vi "Safety_Check.vi"(1 "Adam Loop Count":i32, 2 "Ch Names":string[](array[string]), 3 "Values":dbl[](array[numeric]) format="%.2f") -> (0 "Scan comment":string)   [LabVIEW 2010]
uses:
  ADAM Client/Sub VIs/ADAM Controls/Update_scan_value.ctl
  Anemometry/Anemometry Sub Vis/Globals/Gas_management_global.vi
  ADAM_Global.vi
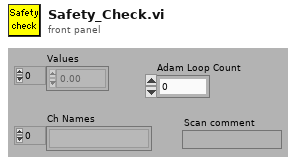
[diagram p1: front panel]
types:
  T1 = cluster{"Channel name":string, "Set value of A to":dbl, "Set value of B to":dbl, "Set value of C to":dbl, "Set value of D to":dbl}
  T2 = typedef "Update_scan_value.ctl" = cluster{"Channel Name":string, "New Value":dbl}
  T3 = enum16{"Append to Global", "Read Global then Clear"}
  T4 = enum16{"On", "Off", "Always On", "Always Off", "Delete"}
  T5 = typedef "LVDateTimeRec.ctl" = cluster{"fractional second":dbl, "second":i32, "minute":i32, "hour":i32, "day of month":i32, "month":i32, "year":i32, "day of week":i32, "day of year":i32, "DST":i32}
  T6 = cluster{"Channel name":string, "Set value of A to":dbl, "Set value of B to":dbl, "Set value of C to":dbl, "Set value of D to":dbl}[]
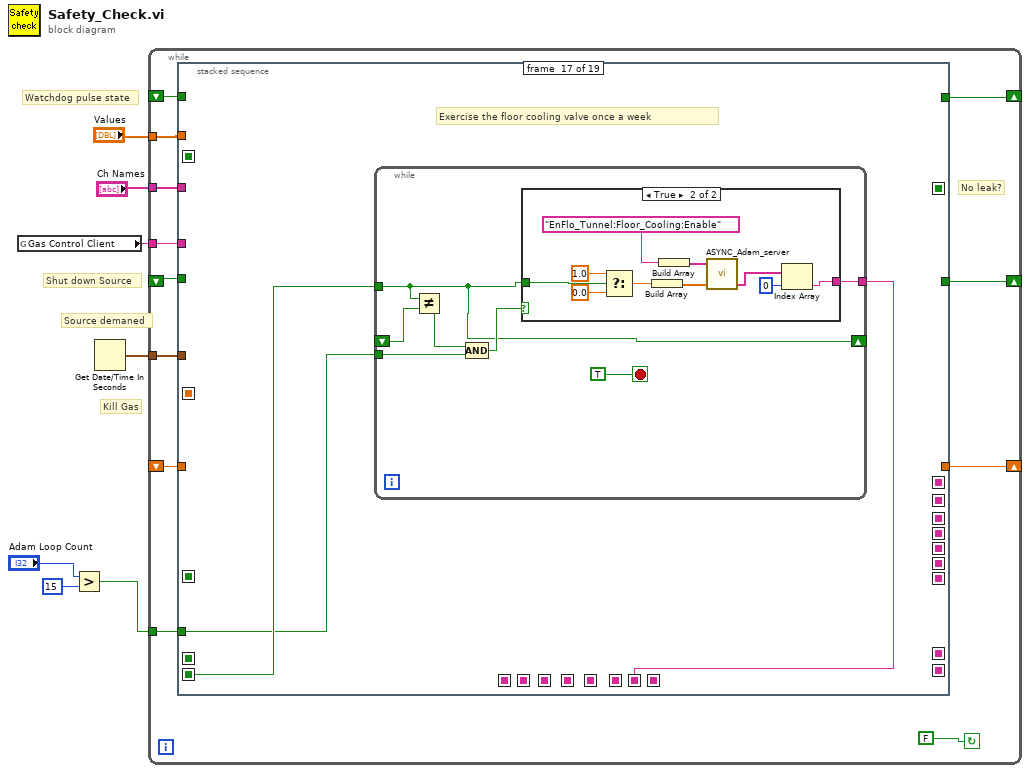
[diagram p0: block diagram]
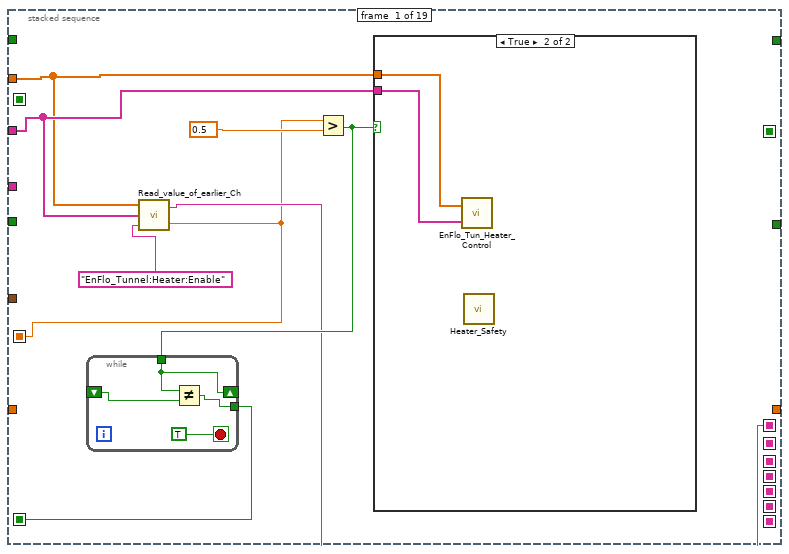
[diagram p2: hidden frame]
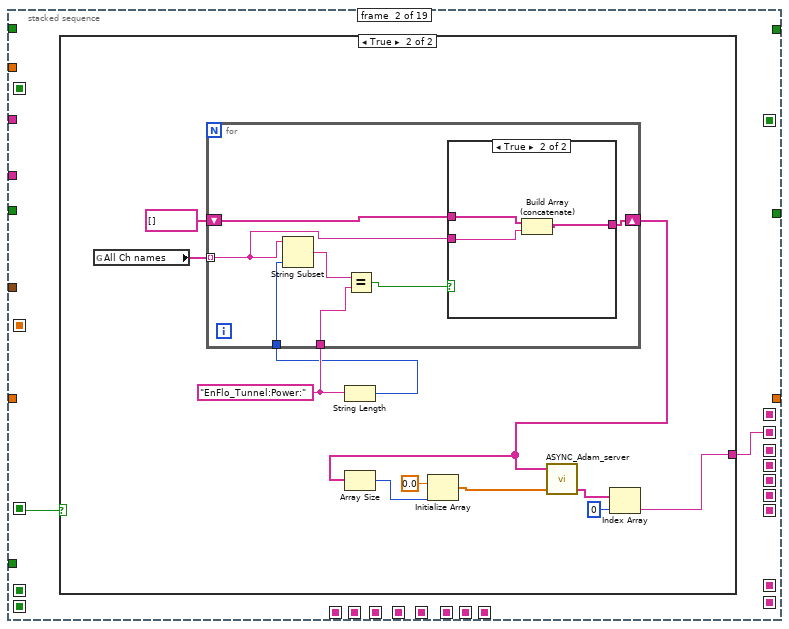
[diagram p4: hidden frame]
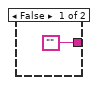
[diagram p5: hidden frame]
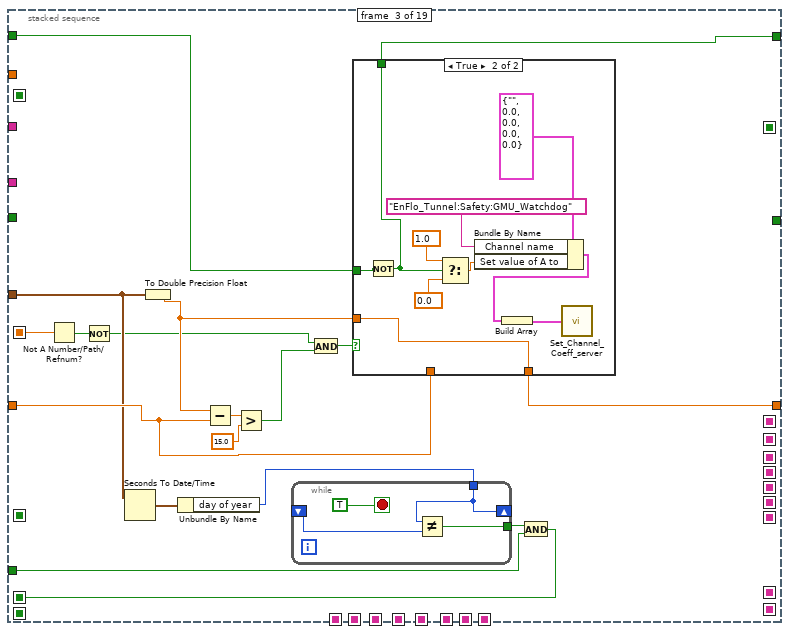
[diagram p7: hidden frame]
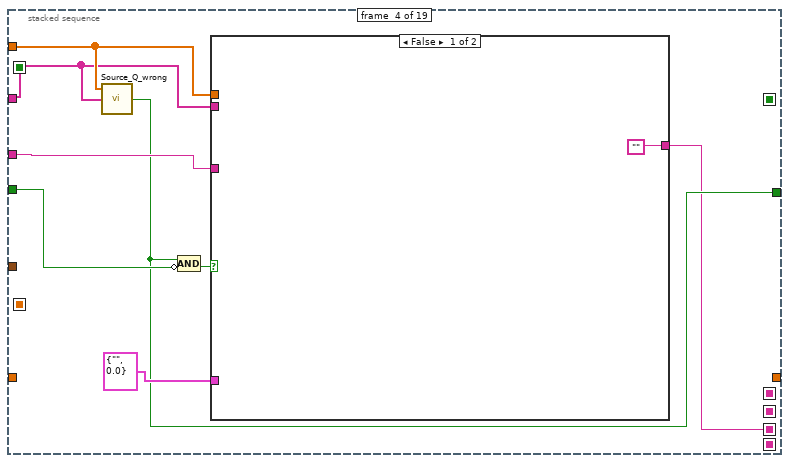
[diagram p9: hidden frame]
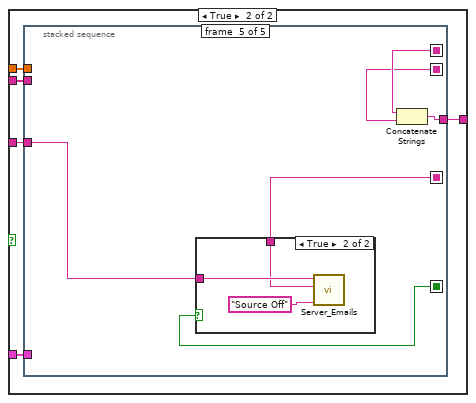
[diagram p10: hidden frame]
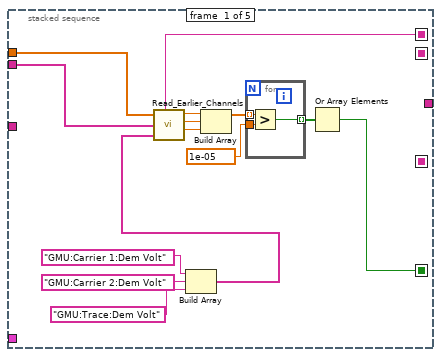
[diagram p11: hidden frame]
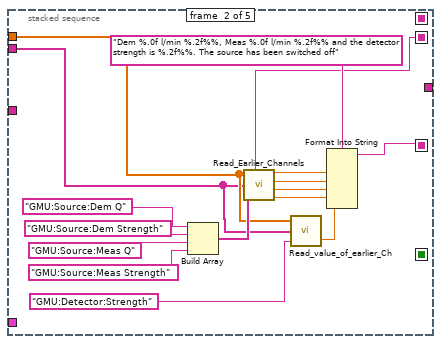
[diagram p12: hidden frame]
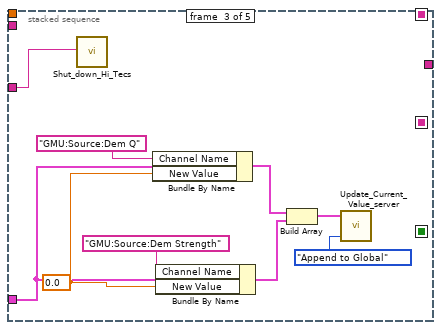
[diagram p13: hidden frame]
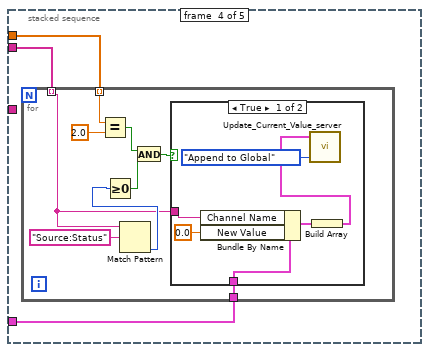
[diagram p14: hidden frame]
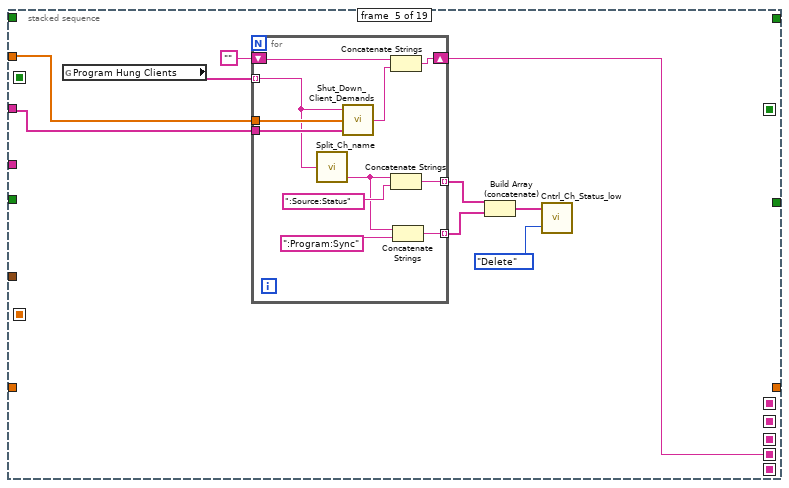
[diagram p17: hidden frame]
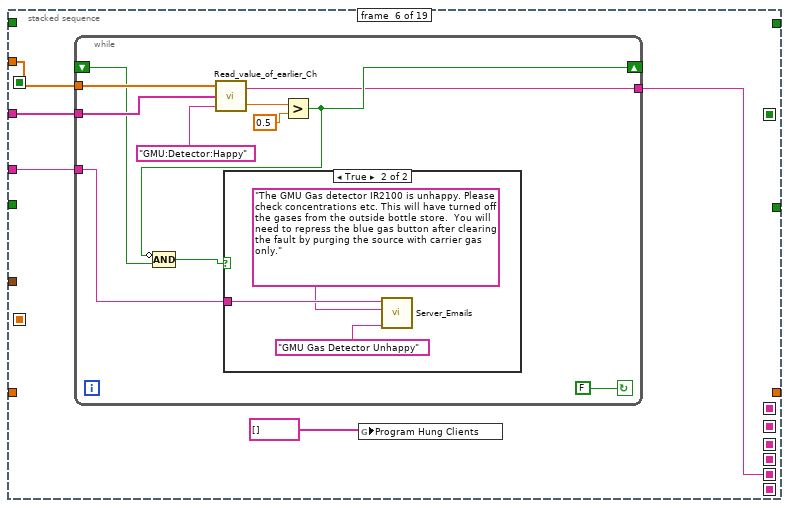
[diagram p18: hidden frame]
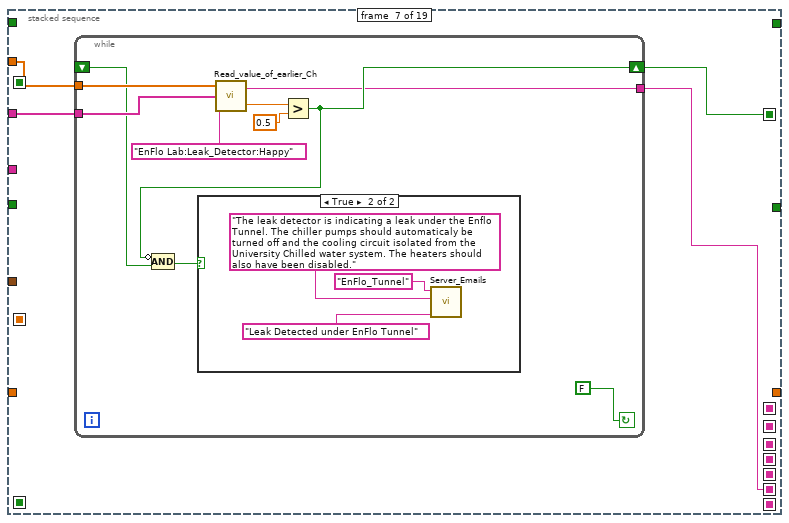
[diagram p20: hidden frame]
diagram:
  # "Shut down Source"
  # "Source demaned"
  # "Watchdog pulse state"
  # "Kill Gas"
  n1 = global read "Gas_management_global.vi" "Gas Control Client"() -> (w5:string)
  n2 = Greater?(x="Adam Loop Count", y=15) -> (0:w2:bool)
  n3 = Get Date/Time In Seconds() -> (seconds since 1Jan1904=w1:timestamp)
  n4 = while {
    shift-left: _ -> [w14]
    shift-right: [w13] -> _
    shift-left: _ -> [w16]
    shift-right: [w15] -> _
    tunnel: w5 -> [w18]
    tunnel: "Ch Names" -> [w19]
    tunnel: "Values" -> [w17]
    shift-right: [w11] -> _
    shift-left: _ -> [w10]
    tunnel: w2 -> [w9]
    tunnel: w1 -> [w8]
    stop <- FALSE continue-if-true
    # "No leak?"
    n5 = stacked-sequence {
      seq-local: [_ _ _ _ _ _ w216 _ _ _ _ _ _ _ _ _ _ _ _] -> [_ _ _ _ _ _ _ _ _ _ w308 _ _ _ _ _ _ _ _]
      seq-local: [w22 _ _ _ _ _ _ _ _ _ _ _ _ _ _ _ _ _ _] -> [_ w35 _ _ _ _ _ _ _ _ _ _ _ _ _ _ _ _ _]
      seq-local: [_ _ w65 _ _ _ _ _ _ _ _ _ _ _ _ _ _ _ _] -> [_ _ _ _ _ _ _ _ _ _ _ _ _ _ _ _ _ _ _]
      seq-local: [_ _ _ _ _ _ _ _ _ _ _ _ w368 _ _ _ _ _ _] -> [_ _ _ _ _ _ _ _ _ _ _ _ _ w386 _ _ _ _ _]
      seq-local: [_ _ _ _ _ _ _ _ _ _ _ _ _ w378 _ _ _ _ _] -> [_ _ _ _ _ _ _ _ _ _ _ _ _ _ _ _ w510 _ _]
      seq-local: [w21 _ _ _ _ _ _ _ _ _ _ _ _ _ _ _ _ _ _] -> [_ _ _ _ _ _ _ _ _ _ _ _ _ _ _ _ _ _ w597]
      seq-local: [_ w34 _ _ _ _ _ _ _ _ _ _ _ _ _ _ _ _ _] -> [_ _ _ _ _ _ _ _ _ _ _ _ _ _ _ _ _ _ w596]
      seq-local: [_ _ _ w93 _ _ _ _ _ _ _ _ _ _ _ _ _ _ _] -> [_ _ _ _ _ _ _ _ _ _ _ _ _ _ _ _ _ _ w595]
      seq-local: [_ _ _ _ w176 _ _ _ _ _ _ _ _ _ _ _ _ _ _] -> [_ _ _ _ _ _ _ _ _ _ _ _ _ _ _ _ _ _ w594]
      seq-local: [_ _ _ _ _ w196 _ _ _ _ _ _ _ _ _ _ _ _ _] -> [_ _ _ _ _ _ _ _ _ _ _ _ _ _ _ _ _ _ w593]
      seq-local: [_ _ _ _ _ _ w215 _ _ _ _ _ _ _ _ _ _ _ _] -> [_ _ _ _ _ _ _ _ _ _ _ _ _ _ _ _ _ _ w592]
      seq-local: [_ _ _ _ _ _ _ w232 _ _ _ _ _ _ _ _ _ _ _] -> [_ _ _ _ _ _ _ _ _ _ _ _ _ _ _ _ _ _ w591]
      seq-local: [_ _ _ _ _ _ _ _ w264 _ _ _ _ _ _ _ _ _ _] -> [_ _ _ _ _ _ _ _ _ _ _ _ _ _ _ _ _ _ w581]
      seq-local: [_ _ _ _ _ _ _ _ _ w284 _ _ _ _ _ _ _ _ _] -> [_ _ _ _ _ _ _ _ _ _ _ _ _ _ _ _ _ _ w580]
      seq-local: [_ _ _ _ _ _ _ _ _ _ w305 _ _ _ _ _ _ _ _] -> [_ _ _ _ _ _ _ _ _ _ _ _ _ _ _ _ _ _ w583]
      seq-local: [_ _ _ _ _ _ _ _ _ _ _ w333 _ _ _ _ _ _ _] -> [_ _ _ _ _ _ _ _ _ _ _ _ _ _ _ _ _ _ w584]
      seq-local: [_ _ _ _ _ _ _ _ _ _ _ _ w356 _ _ _ _ _ _] -> [_ _ _ _ _ _ _ _ _ _ _ _ _ _ _ _ _ _ w585]
      seq-local: [_ _ _ _ _ _ _ _ _ _ _ _ _ w375 _ _ _ _ _] -> [_ _ _ _ _ _ _ _ _ _ _ _ _ _ _ _ _ _ w586]
      seq-local: [_ _ _ _ _ _ _ _ _ _ _ _ _ _ w443 _ _ _ _] -> [_ _ _ _ _ _ _ _ _ _ _ _ _ _ _ _ _ _ w587]
      seq-local: [_ _ _ _ _ _ _ _ _ _ _ _ _ _ _ w472 _ _ _] -> [_ _ _ _ _ _ _ _ _ _ _ _ _ _ _ _ _ _ w588]
      seq-local: [_ _ _ _ _ _ _ _ _ _ _ _ _ _ _ _ w508 _ _] -> [_ _ _ _ _ _ _ _ _ _ _ _ _ _ _ _ _ _ w589]
      seq-local: [_ _ _ _ _ _ _ _ _ _ _ _ _ _ _ _ _ w529 _] -> [_ _ _ _ _ _ _ _ _ _ _ _ _ _ _ _ _ _ w590]
      seq-local: [w20 _ _ _ _ _ _ _ _ _ _ _ _ _ _ _ _ _ _] -> [_ _ w63 _ _ _ _ _ _ _ _ _ _ _ _ _ _ _ _]
      tunnel: w19 -> [w25 _ _ w95 w183 w198 w217 w233 w265 w286 w306 w339 w364 w387 w448 w475 _ w536 _]
      tunnel: w18 -> [_ _ _ w100 _ w197 _ _ _ _ _ _ _ _ _ _ _ _ _]
      tunnel: w17 -> [w24 _ _ w96 w179 w199 w218 w234 w266 w287 w307 w340 w365 w388 w449 w476 _ w535 _]
      tunnel: w16 -> [_ _ w76 _ _ _ _ _ _ _ _ _ _ _ _ _ _ _ _]
      tunnel: [_ _ w75 _ _ _ _ _ _ _ _ _ _ _ _ _ _ _ _] -> w15
      tunnel: w14 -> [_ _ _ w99 _ _ _ _ _ _ _ _ _ _ _ _ _ _ _]
      tunnel: [_ _ _ w94 _ _ _ _ _ _ _ _ _ _ _ _ _ _ _] -> w13
      tunnel: [_ _ w74 _ _ _ _ _ _ _ _ _ _ _ _ _ _ _ _] -> w11
      tunnel: w10 -> [_ _ w70 _ _ _ _ _ _ _ _ _ _ _ _ _ _ _ _]
      tunnel: w9 -> [_ _ w66 _ _ _ _ _ _ w285 _ _ _ w379 w444 _ w509 w530 _]
      tunnel: w8 -> [_ _ w64 _ _ _ _ _ _ _ _ _ _ _ _ _ _ _ _]
      frame #0 {
        n6 = call "Read_value_of_earlier_Ch.vi"("Desired Ch to Read"="EnFlo_Tunnel:Heater:Enable", "Ch names"=w25, "Present scan array"=w24) -> ("Value"=w20:dbl, "Scan comment"=w21:string)  [unwired: 1 in]
        n7 = Greater?(x=w20, y=0.5) -> (0:w23:bool)
        n8 = while {
          shift-right: [w31] -> _
          shift-left: _ -> [w30]
          tunnel: w23 -> [w31]
          tunnel: [w28] -> w22
          stop <- TRUE stop-if-true
          n9 = Not Equal?(x=w31, y=w30) -> (x != y?=w28:bool)
        }
        n10 = case shown="True" w23 {
          tunnel: w24 -> [_ w33]
          tunnel: w25 -> [_ w32]
          frame False {
          }
          frame True {
            n11 = call "EnFlo_Tun_Heater_Control.vi"("Ch Names"=w32, "Values"=w33) -> ()  [unwired: 1 out]
            n12 = call "Heater_Safety.vi"() -> ()  [unwired: 3 in, 5 out]
          }
        }
      }
      frame #1 {
        n13 = case shown="True" w35 {
          tunnel: ["" w38] -> w34
          frame False {
          }
          frame True {
            w47 = "EnFlo_Tunnel:Power:"
            n14 = global read "ADAM_Global.vi" "All Ch names"() -> (w37:string[])
            n15 = String Length(string=w47) -> (length=w46:i32)
            n16 = for {
              shift-right: [w49] -> w42
              shift-left: string[] [] -> [w50]
              tunnel: w37 -> [w53] mode=indexing
              tunnel: w46 -> [w54]
              tunnel: w47 -> [w51]
              n17 = String Subset(string=w53, length (rest)=w54) -> (substring=w52:string)  [unwired: 1 out]
              n18 = Equal?(x=w52, y=w51) -> (x = y?=w48:bool)
              n19 = case shown="True" w48 {
                tunnel: w53 -> [_ w58]
                tunnel: w50 -> [w55 w56]
                tunnel: [w55 w57] -> w49
                frame False {
                }
                frame True {
                  n20 = Build Array (concatenate)(w56, w58) -> (w57:string[])
                }
              }
            }
            n21 = Array Size(array=w42) -> (size(s)=w43:i32)
            n22 = Initialize Array(0.0 ("element"), w43) -> (w41:dbl[])
            n23 = call "ASYNC_Adam_server.vi"("Values"=w41, "Channel Names"=w42) -> ("Scan Comments"=w40:string[])  [unwired: 1 in, 2 out]
            n24 = Index Array(array=w40, index=0) -> (element=w38:string)
          }
        }
      }
      frame #2 {
        n25 = Not A Number/Path/Refnum?(number/path/refnum=w63) -> (NaN/Path/Refnum?=w62:bool)
        n26 = Not(x=w62) -> (.not. x?=w60:bool)
        n27 = Seconds To Date/Time(time stamp (now)=w64) -> (date time rec=w69:T5)  [unwired: 1 in]
        n28 = To Double Precision Float(number=w64) -> (double precision float=w73:dbl)
        n29 = Unbundle By Name(w69) -> ("day of year"=w68:i32)
        n30 = Subtract(x=w73, y=w70) -> (x-y=w72:dbl)
        n31 = Greater?(x=w72, y=15.0) -> (0:w61:bool)
        n32 = while {
          shift-right: [w80] -> _
          shift-left: _ -> [w79]
          tunnel: w68 -> [w80]
          tunnel: [w78] -> w67
          stop <- TRUE stop-if-true
          n33 = Not Equal?(x=w80, y=w79) -> (x != y?=w78:bool)
        }
        n34 = And(x=w60, y=w61) -> (x .and. y?=w59:bool)
        n35 = case shown="True" w59 {
          tunnel: w76 -> [w81 w85]
          tunnel: [w81 w84] -> w75
          tunnel: [w82 w83] -> w74
          tunnel: w73 -> [_ w83]
          tunnel: w70 -> [w82 _]
          frame False {
          }
          frame True {
            n36 = Not(x=w85) -> (.not. x?=w84:bool)
            n37 = Select(t=1.0 ("Suction"), s=w84, f=0.0 ("Suction")) -> (s? t:f=w88:dbl)
            n38 = Bundle By Name(cluster=T1 {"Channel name"="", "Set value of A to"=0.0, "Set value of B to"=0.0, "Set value of C to"=0.0, "Set value of D to"=0.0}, "Channel name"="EnFlo_Tunnel:Safety:GMU_Watchdog" ("Desired Ch to Read"), "Set value of A to"=w88) -> (w92:T1)
            n39 = Build Array(w92) -> (w87:T6)
            n40 = call "Set_Channel_Coeff_server.vi"("Set Array"=w87) -> ()
          }
        }
        n41 = And(x=w67, y=w66) -> (x .and. y?=w65:bool)
      }
      frame #3 {
        n42 = call "Source_Q_wrong.vi"("Ch Names"=w95, "Values"=w96) -> ("Gas Error?"=w94:bool)  [unwired: 1 out]
        n43 = Compound Arithmetic op=AND(w94, invert w99) -> (w98:bool)
        n44 = case shown="False" w98 {
          tunnel: w100 -> [_ w106]
          tunnel: w96 -> [_ w105]
          tunnel: w95 -> [_ w104]
          tunnel: T2 {"Channel Name"="", "New Value"=0.0} ("Update Scan Value Cluster") -> [_ w103]
          tunnel: ["" w102] -> w93
          frame False {
          }
          frame True {
            n45 = stacked-sequence {
              seq-local: [_ w138 _ _ _] -> [_ _ _ _ w171]
              seq-local: [w108 _ _ _ _] -> [_ _ _ _ w170]
              seq-local: [w107 _ _ _ _] -> [_ _ _ _ w169]
              seq-local: [_ w124 _ _ _] -> [_ _ _ _ w168]
              tunnel: w106 -> [_ _ w141 _ w172]
              tunnel: w105 -> [w118 w128 _ w150 _]
              tunnel: w104 -> [w119 w127 _ w151 _]
              tunnel: w103 -> [_ _ w140 w149 _]
              tunnel: [_ _ _ _ w167] -> w102
              frame #0 {
                n46 = Build Array("GMU:Carrier 1:Dem Volt", "GMU:Carrier 2:Dem Volt", "GMU:Trace:Dem Volt") -> (w120:string[])
                n47 = call "Read_Earlier_Channels.vi"("Present scan array"=w118, "Ch names"=w119, "Desired Channels"=w120) -> ("Scan comments"=w107:string, "Index 0"=w114:dbl, "Index 1"=w113:dbl, "Index 2"=w112:dbl)  [unwired: 2 out]
                n48 = Build Array(w114, w113, w112) -> (w111:dbl[])
                n49 = for {
                  tunnel: w111 -> [w123] mode=indexing
                  tunnel: 1e-05 -> [w122]
                  tunnel: [w121] -> w109 mode=indexing
                  n50 = Greater?(x=w123, y=w122) -> (0:w121:bool)
                }
                n51 = Or Array Elements(Boolean array=w109) -> (logical OR=w108:bool)
              }
              frame #1 {
                n52 = Build Array("GMU:Source:Dem Q", "GMU:Source:Dem Strength", "GMU:Source:Meas Q", "GMU:Source:Meas Strength") -> (w133:string[])
                n53 = call "Read_Earlier_Channels.vi"("Present scan array"=w128, "Ch names"=w127, "Desired Channels"=w133) -> ("Scan comments"=w124:string, "Index 0"=w132:dbl, "Index 1"=w131:dbl, "Index 2"=w130:dbl, "Index 3"=w129:dbl)  [unwired: 1 out]
                n54 = call "Read_value_of_earlier_Ch.vi"("Desired Ch to Read"="GMU:Detector:Strength", "Ch names"=w127, "Present scan array"=w128) -> ("Value"=w125:dbl)  [unwired: 1 in, 1 out]
                n55 = Format Into String(format string="Dem %.0f l/min %.2f%%, Meas %.0f l/min %.2f%% and the detector strength is %.2f%%. The source has been switched off" ("Format String"), w132, w131, w130, w129, w125) -> (resulting string=w138:string)  [unwired: 2 in, 1 out]
              }
              frame #2 {
                w142 = 0.0 ("Bundle Element")
                n56 = call "Shut_down_Hi_Tecs.vi"("Client Name"=w141) -> ()  [unwired: 6 out]
                n57 = Bundle By Name(cluster=w140, "Channel Name"="GMU:Source:Dem Q", "New Value"=w142) -> (w147:T2)
                n58 = Bundle By Name(cluster=w140, "Channel Name"="GMU:Source:Dem Strength", "New Value"=w142) -> (w148:T2)
                n59 = Build Array(w147, w148) -> (w144:T2[])
                n60 = call "Update_Current_Value_server.vi"("Mode"=T3."Append to Global", "Update array in"=w144) -> ()  [unwired: 1 in, 1 out]
              }
              frame #3 {
                n61 = for {
                  tunnel: w151 -> [w152] mode=indexing
                  tunnel: w150 -> [w158] mode=indexing
                  tunnel: w149 -> [w153]
                  n62 = Equal?(x=w158, y=2.0) -> (x = y?=w155:bool)
                  n63 = Match Pattern(string=w152, regular expression="Source:Status") -> (offset past match=w159:i32)  [unwired: 4 out]
                  n64 = Greater Or Equal To 0?(x=w159) -> (x >= 0?=w156:bool)
                  n65 = And(x=w155, y=w156) -> (x .and. y?=w154:bool)
                  n66 = case shown="True" w154 {
                    tunnel: w153 -> [w166 _]
                    tunnel: w152 -> [w165 _]
                    frame True {
                      n67 = Bundle By Name(cluster=w166, "Channel Name"=w165, "New Value"=0.0) -> (w163:T2)
                      n68 = Build Array(w163) -> (w162:T2[])
                      n69 = call "Update_Current_Value_server.vi"("Mode"=T3."Append to Global", "Update array in"=w162) -> ()  [unwired: 1 in, 1 out]
                    }
                    frame False {
                    }
                  }
                }
              }
              frame #4 {
                n70 = case shown="True" w170 {
                  tunnel: w172 -> [_ w175]
                  tunnel: w171 -> [_ w174]
                  frame False {
                  }
                  frame True {
                    n71 = call "Server_Emails.vi"("Client Name Contains"=w175, "Message"=w174, "Subject"="Source Off") -> ()  [unwired: 2 in, 3 out]
                  }
                }
                n72 = Concatenate Strings(w169, w168) -> (w167:string)
              }
            }
          }
        }
      }
      frame #4 {
        n73 = global read "ADAM_Global.vi" "Program Hung Clients"() -> (w184:string[])
        n74 = for {
          tunnel: w184 -> [w193] mode=indexing
          tunnel: w179 -> [w195]
          tunnel: w183 -> [w194]
          tunnel: [w191] -> w182 mode=indexing
          tunnel: [w188] -> w181 mode=indexing
          shift-right: [w186] -> w176
          shift-left: "" -> [w187]
          n75 = call "Split_Ch_name.vi"("Ch name"=w193) -> ("Low level"=w190:string)  [unwired: 2 out]
          n76 = call "Shut_Down_Client_Demands.vi"("Ch Names"=w194, "Values"=w195, "Client Name"=w193) -> ("Comments"=w185:string)
          n77 = Concatenate Strings(w187, w185) -> (w186:string)
          n78 = Concatenate Strings(w190, ":Source:Status") -> (w191:string)
          n79 = Concatenate Strings(w190, ":Program:Sync") -> (w188:string)
        }
        n80 = Build Array (concatenate)(w182, w181) -> (w180:string[])
        n81 = call "Cntrl_Ch_Status_low.vi"("Mode"=T4."Delete", "Channel names"=w180) -> ()  [unwired: 1 out]
      }
      frame #5 {
        n82 = while {
          tunnel: w199 -> [w211]
          tunnel: w198 -> [w210]
          shift-right: [w205] -> _
          shift-left: _ -> [w206]
          tunnel: w197 -> [w203]
          tunnel: [w201] -> w196
          stop <- FALSE continue-if-true
          n83 = call "Read_value_of_earlier_Ch.vi"("Desired Ch to Read"="GMU:Detector:Happy", "Ch names"=w210, "Present scan array"=w211) -> ("Value"=w208:dbl, "Scan comment"=w201:string)  [unwired: 1 in]
          n84 = Greater?(x=w208, y=0.5) -> (0:w205:bool)
          n85 = Compound Arithmetic op=AND(invert w205, w206) -> (w204:bool)
          n86 = case shown="True" w204 {
            tunnel: w203 -> [_ w213]
            frame False {
            }
            frame True {
              n87 = call "Server_Emails.vi"("Client Name Contains"=w213, "Message"="The GMU Gas detector IR2100 is unhappy. Please check concentrations etc. This will have turned off the gases from the outside bottle store.  You will need to repress the blue gas button after clearing the fault by purging the source with carrier gas only.", "Subject"="GMU Gas Detector Unhappy") -> ()  [unwired: 2 in, 3 out]
            }
          }
        }
        n88 = global write "ADAM_Global.vi" "Program Hung Clients"(string[] [] ("Program Hung Clients")) -> ()
      }
      frame #6 {
        n89 = while {
          tunnel: w218 -> [w228]
          tunnel: w217 -> [w227]
          shift-right: [w222] -> w216
          shift-left: _ -> [w223]
          tunnel: [w219] -> w215
          stop <- FALSE continue-if-true
          n90 = call "Read_value_of_earlier_Ch.vi"("Desired Ch to Read"="EnFlo Lab:Leak_Detector:Happy", "Ch names"=w227, "Present scan array"=w228) -> ("Value"=w225:dbl, "Scan comment"=w219:string)  [unwired: 1 in]
          n91 = Greater?(x=w225, y=0.5) -> (0:w222:bool)
          n92 = Compound Arithmetic op=AND(invert w222, w223) -> (w221:bool)
          n93 = case shown="True" w221 {
            frame False {
            }
            frame True {
              n94 = call "Server_Emails.vi"("Client Name Contains"="EnFlo_Tunnel", "Message"="The leak detector is indicating a leak under the Enflo Tunnel. The chiller pumps should automaticaly be turned off and the cooling circuit isolated from the  University Chilled water system. The heaters should also have been disabled.", "Subject"="Leak Detected under EnFlo Tunnel") -> ()  [unwired: 2 in, 3 out]
            }
          }
        }
      }
      frame #7 {
        n95 = while {
          tunnel: w234 -> [w250]
          tunnel: w233 -> [w249]
          shift-right: [w243] -> _
          shift-left: _ -> [w239]
          tunnel: [w235] -> w232
          stop <- FALSE continue-if-true
          w241 = 60.0 ("y")
          n96 = Decrement(x=w241) -> (x-1=w242:dbl)
          n97 = Select(t=w242, s=w239, f=w241) -> (s? t:f=w240:dbl)
          n98 = call "Read_value_of_earlier_Ch.vi"("Desired Ch to Read"="EnFlo_Tunnel:Chilled Water:Motor1 Temp", "Ch names"=w249, "Present scan array"=w250) -> ("Value"=w257:dbl, "Scan comment"=w237:string)  [unwired: 1 in]
          n99 = call "Read_value_of_earlier_Ch.vi"("Desired Ch to Read"="EnFlo_Tunnel:Chilled Water:Motor2 Temp", "Ch names"=w249, "Present scan array"=w250) -> ("Value"=w254:dbl, "Scan comment"=w236:string)  [unwired: 1 in]
          n100 = Greater?(x=w257, y=w240) -> (0:w251:bool)
          n101 = Greater?(x=w254, y=w240) -> (0:w252:bool)
          n102 = Or(x=w251, y=w252) -> (x .or. y?=w245:bool)
          n103 = call "Read_value_of_earlier_Ch.vi"("Desired Ch to Read"="EnFlo_Tunnel:Chiller_Pump:Enable", "Ch names"=w249, "Present scan array"=w250) -> ("Value"=w247:dbl, "Scan comment"=w238:string)  [unwired: 1 in]
          n104 = Greater?(x=w247, y=0.5) -> (0:w244:bool)
          n105 = And(x=w244, y=w245) -> (x .and. y?=w243:bool)
          n106 = Compound Arithmetic op=AND(w243, invert w239) -> (w256:bool)
          n107 = case shown="False" w256 {
            tunnel: w241 -> [_ w260]
            frame False {
            }
            frame True {
              n108 = Format Into String(format string="The Chilled Water Motor Temp is greater than %.0f deg C." ("Message"), w260) -> (resulting string=w259:string)  [unwired: 2 in, 1 out]
              n109 = call "Server_Emails.vi"("Client Name Contains"="EnFlo_Tunnel", "Message"=w259, "Subject"="Chilled Water Motor Temp") -> ()  [unwired: 2 in, 3 out]
            }
          }
          n110 = Concatenate Strings(w238, w237, w236) -> (w235:string)
        }
      }
      frame #8 {
        n111 = while {
          tunnel: w266 -> [w280]
          tunnel: w265 -> [w279]
          shift-right: [w268] -> _
          shift-left: _ -> [w274]
          shift-left: _ -> [w273]
          shift-left: _ -> [w272]
          tunnel: [w267] -> w264
          stop <- FALSE continue-if-true
          n112 = call "Read_value_of_earlier_Ch.vi"("Desired Ch to Read"="FFID:System:Enable", "Ch names"=w279, "Present scan array"=w280) -> ("Value"=w275:dbl, "Scan comment"=w267:string)  [unwired: 1 in]
          n113 = Greater?(x=w275, y=0.5) -> (0:w268:bool)
          n114 = Compound Arithmetic op=AND(w268, w274, invert w273, invert w272) -> (w270:bool)
          n115 = Compound Arithmetic op=AND(invert w268, invert w274, w273, w272) -> (w271:bool)
          n116 = Or(x=w270, y=w271) -> (x .or. y?=w269:bool)
          n117 = case shown="True" w269 {
            tunnel: w275 -> [_ w281]
            tunnel: w268 -> [_ _]
            frame False {
            }
            frame True {
              n118 = Build Array(w281) -> (w283:dbl[])
              n119 = call "ASYNC_Adam_server.vi"("Values"=w283, "Channel Names"=string[] ["GMU:Gas:Enable"]) -> ()  [unwired: 1 in, 3 out]
            }
          }
        }
      }
      frame #9 {
        # "Resetting A Tunnel speed to zero if the drive in turned off\nso that the belts do not slip when the tunnel is turned on again."
        n120 = while {
          tunnel: w287 -> [w300]
          tunnel: w286 -> [w299]
          shift-right: [w291] -> _
          shift-left: _ -> [w294]
          shift-left: _ -> [w293]
          shift-left: _ -> [w292]
          tunnel: w285 -> [w290]
          tunnel: [w288] -> w284
          stop <- FALSE continue-if-true
          n121 = call "Read_value_of_earlier_Ch.vi"("Desired Ch to Read"="A_Tunnel:Motor:Enable", "Ch names"=w299, "Present scan array"=w300) -> ("Value"=w295:dbl, "Scan comment"=w288:string)  [unwired: 1 in]
          n122 = Less?(x=w295, y=0.5) -> (x < y?=w291:bool)
          n123 = Compound Arithmetic op=AND(w291, w294, invert w293, invert w292, w290) -> (w289:bool)
          n124 = case shown="True" w289 {
            tunnel: w291 -> [_ _]
            frame False {
            }
            frame True {
              w303 = string[] ["A_Tunnel:Speed:Dem Velocity", "A_Tunnel:Speed:Dem Voltage"] ("Channel Names")
              n125 = Array Size(array=w303) -> (size(s)=w304:i32)
              n126 = Initialize Array(0.0 ("element"), w304) -> (w302:dbl[])
              n127 = call "ASYNC_Adam_server.vi"("Values"=w302, "Channel Names"=w303) -> ()  [unwired: 1 in, 3 out]
            }
          }
        }
      }
      frame #10 {
        n128 = case shown="True" w308 {
          tunnel: w307 -> [w313 _]
          tunnel: w306 -> [w312 _]
          tunnel: [w309 ""] -> w305
          frame False {
            n129 = for {
              tunnel: w313 -> [w323]
              tunnel: w312 -> [w322]
              tunnel: string[] ["EnFlo_Tunnel:Heater:Enable", "EnFlo_Tunnel:Chiller_Pump:Enable", "EnFlo_Tunnel:Tap_Water:Enable"] ("Ch Names") -> [w318] mode=indexing
              shift-right: [w316] -> w309
              shift-left: "" -> [w317]
              n130 = call "Read_value_of_earlier_Ch.vi"("Desired Ch to Read"=w318, "Ch names"=w322, "Present scan array"=w323) -> ("Value"=w320:dbl, "Scan comment"=w315:string)  [unwired: 1 in]
              n131 = Greater?(x=w320, y=0.5) -> (0:w319:bool)
              n132 = case shown="False" w319 {
                tunnel: w318 -> [_ w328]
                tunnel: ["" w325] -> w314
                frame False {
                }
                frame True {
                  n133 = Build Array(w328) -> (w331:string[])
                  n134 = Build Array(0.0) -> (w330:dbl[])
                  n135 = call "ASYNC_Adam_server.vi"("Values"=w330, "Channel Names"=w331) -> ("Scan Comments"=w326:string[])  [unwired: 1 in, 2 out]
                  n136 = Index Array(array=w326, index=0) -> (element=w325:string)
                }
              }
              n137 = Concatenate Strings(w317, w315, w314) -> (w316:string)
            }
          }
          frame True {
          }
        }
      }
      frame #11 {
        w341 = "EnFlo_Tunnel:Heater:Enable" ("Ch Name")
        n138 = call "Read_value_of_earlier_Ch.vi"("Desired Ch to Read"=w341, "Ch names"=w339, "Present scan array"=w340) -> ("Value"=w346:dbl, "Scan comment"=w335:string)  [unwired: 1 in]
        n139 = call "Read_value_of_earlier_Ch.vi"("Desired Ch to Read"="EnFlo_Tunnel:Reference:Velocity", "Ch names"=w339, "Present scan array"=w340) -> ("Value"=w343:dbl, "Scan comment"=w334:string)  [unwired: 1 in]
        n140 = Greater?(x=w346, y=0.5) -> (0:w338:bool)
        n141 = Less?(x=w343, y=0.25) -> (x < y?=w342:bool)
        n142 = And(x=w338, y=w342) -> (x .and. y?=w337:bool)
        n143 = case shown="False" w337 {
          tunnel: w341 -> [_ w352]
          tunnel: ["" w349] -> w336
          frame False {
          }
          frame True {
            n144 = Build Array(w352) -> (w355:string[])
            n145 = Build Array(0.0) -> (w354:dbl[])
            n146 = call "ASYNC_Adam_server.vi"("Values"=w354, "Channel Names"=w355) -> ("Scan Comments"=w350:string[])  [unwired: 1 in, 2 out]
            n147 = Index Array(array=w350, index=0) -> (element=w349:string)
          }
        }
        n148 = Concatenate Strings(w335, w334, w336) -> (w333:string)
      }
      frame #12 {
        n149 = call "Read_value_of_earlier_Ch.vi"("Desired Ch to Read"="EnFlo_Tunnel:Chiller_Pump:Running", "Ch names"=w364, "Present scan array"=w365) -> ("Value"=w366:dbl, "Scan comment"=w359:string)  [unwired: 1 in]
        n150 = call "Read_value_of_earlier_Ch.vi"("Desired Ch to Read"="Uni:Chilled Water:Temp", "Ch names"=w364, "Present scan array"=w365) -> ("Value"=w361:dbl, "Scan comment"=w358:string)  [unwired: 1 in]
        n151 = call "Read_value_of_earlier_Ch.vi"("Desired Ch to Read"="EnFlo_Tunnel:Reference:Velocity", "Ch names"=w364, "Present scan array"=w365) -> ("Value"=w360:dbl, "Scan comment"=w357:string)  [unwired: 1 in]
        n152 = Less?(x=w361, y=20.0) -> (x < y?=w371:bool)
        n153 = Greater?(x=w360, y=0.4) -> (0:w372:bool)
        n154 = Greater?(x=w366, y=0.5) -> (0:w374:bool)
        n155 = Compound Arithmetic op=AND(w374, w371, w372) -> (w368:bool)
        n156 = Concatenate Strings(w359, w358, w357) -> (w356:string)
      }
      frame #13 {
        w384 = "EnFlo_Tunnel:Heat_Ex_Div_Valve:Dem Pos"
        n157 = case shown="False" w386 {
          tunnel: w388 -> [_ w426]
          tunnel: w387 -> [_ w427]
          tunnel: w384 -> [_ w430]
          tunnel: [0.0 ("upper limit") w436] -> w380
          tunnel: ["" w421] -> w377
          frame False {
          }
          frame True {
            n158 = call "Read_value_of_earlier_Ch.vi"("Desired Ch to Read"="EnFlo_Tunnel:Exit Duct:Dem Temp", "Ch names"=w427, "Present scan array"=w426) -> ("Value"=w435:dbl, "Scan comment"=w425:string)  [unwired: 1 in]
            n159 = call "Read_value_of_earlier_Ch.vi"("Desired Ch to Read"="EnFlo_Tunnel:Exit Duct Top:Temp", "Ch names"=w427, "Present scan array"=w426) -> ("Value"=w431:dbl, "Scan comment"=w424:string)  [unwired: 1 in]
            n160 = call "Read_value_of_earlier_Ch.vi"("Desired Ch to Read"="EnFlo_Tunnel:Exit Duct:Temp", "Ch names"=w427, "Present scan array"=w426) -> ("Value"=w432:dbl, "Scan comment"=w423:string)  [unwired: 1 in]
            n161 = call "Read_value_of_earlier_Ch.vi"("Desired Ch to Read"=w430, "Ch names"=w427, "Present scan array"=w426) -> ("Value"=w433:dbl, "Scan comment"=w422:string)  [unwired: 1 in]
            n162 = Add(x=w431, y=w432) -> (x+y=w440:dbl)
            n163 = Divide(x=w440, y=2.0) -> (x/y=w442:dbl)
            n164 = Concatenate Strings(w425, w424, w423, w422) -> (w421:string)
            n165 = call "Back_End_Chiller_PID.vi"("Present Value"=w442, "Previous Control Sum"=w433, "Setpoint"=w435) -> ("Dem Output"=w439:dbl)
            n166 = In Range and Coerce(upper limit=100.0, x=w439, lower limit=0.0) -> (coerced(x)=w436:dbl)  [unwired: 1 out]
          }
        }
        n167 = while {
          shift-right: [w418] -> w385
          shift-left: _ -> [_]
          tunnel: w386 -> [w418]
          shift-left: _ -> [_]
          shift-left: _ -> [_]
          shift-left: _ -> [_]
          shift-left: _ -> [_]
          shift-left: _ -> [_]
          shift-left: _ -> [_]
          shift-left: _ -> [_]
          shift-left: _ -> [_]
          shift-left: _ -> [_]
          shift-left: _ -> [_]
          shift-left: _ -> [_]
          shift-left: _ -> [_]
          shift-left: _ -> [_]
          shift-left: _ -> [_]
          shift-left: _ -> [_]
          shift-left: _ -> [_]
          shift-left: _ -> [w417]
          tunnel: [w417] -> w383
          stop <- TRUE stop-if-true
        }
        n168 = And(x=w385, y=w383) -> (x .and. y?=w382:bool)
        n169 = case shown="False" w382 {
          tunnel: [w390 w401] -> w381
          tunnel: w380 -> [_ w401]
          tunnel: [w389 FALSE] -> w378
          frame False {
            # "Exercise valve once a week"
            n170 = Seconds To Date/Time() -> (date time rec=w391:T5)  [unwired: 2 out]
            n171 = Unbundle By Name(w391) -> ("day of week"=w396:i32, "hour"=w394:i32)
            n172 = Less?(x=w394, y=3) -> (x < y?=w399:bool)
            n173 = Equal?(x=7, y=w396) -> (x = y?=w398:bool)
            n174 = And(x=w398, y=w399) -> (x .and. y?=w389:bool)
            n175 = Select(t=100.0, s=w389, f=0.0) -> (s? t:f=w390:dbl)
          }
          frame True {
          }
        }
        n176 = while {
          shift-right: [w407] -> _
          shift-left: _ -> [w408]
          tunnel: w381 -> [w407]
          tunnel: w384 -> [w409]
          tunnel: w379 -> [w404]
          tunnel: [w402] -> w376
          stop <- TRUE stop-if-true
          n177 = Not Equal?(x=w407, y=w408) -> (x != y?=w405:bool)
          n178 = Compound Arithmetic op=OR(w405, invert w404) -> (w403:bool)
          n179 = Build Array(w409) -> (w410:string[])
          n180 = Build Array(w407) -> (w411:dbl[])
          n181 = case shown="False" w403 {
            tunnel: w411 -> [_ w415]
            tunnel: w410 -> [_ w414]
            tunnel: [string[] [] ("Scan Comments") w413] -> w402
            frame False {
            }
            frame True {
              n182 = call "ASYNC_Adam_server.vi"("Values"=w415, "Channel Names"=w414) -> ("Scan Comments"=w413:string[])  [unwired: 1 in, 2 out]
            }
          }
        }
        n183 = Concatenate Strings(w377, w376) -> (w375:string)
      }
      frame #14 {
        n184 = Search 1D Array(1D array=w448, element="Status:of:EnFlo_Tunnel") -> (index of element=w451:i32)  [unwired: 1 out]
        n185 = Index Array(array=w449, index=w451) -> (element=w447:dbl)
        n186 = case shown="0, Default" w447 {
          tunnel: [0.0 1.0 1.0 1.0] -> w446
          frame 0, Default {
          }
          frame 1 {
          }
          frame 2 {
          }
          frame 3 {
          }
        }
        n187 = while {
          shift-right: [w461] -> _
          shift-left: _ -> [w462]
          tunnel: w446 -> [w461]
          tunnel: "EnFlo_Tunnel:Warning_Cone:Enable" -> [w463]
          tunnel: w444 -> [w458]
          tunnel: [w456] -> w443
          stop <- TRUE stop-if-true
          n188 = Not Equal?(x=w461, y=w462) -> (x != y?=w459:bool)
          n189 = Build Array(w463) -> (w464:string[])
          n190 = Build Array(w461) -> (w465:dbl[])
          n191 = Compound Arithmetic op=OR(w459, invert w458) -> (w457:bool)
          n192 = case shown="False" w457 {
            tunnel: w465 -> [_ w471]
            tunnel: w464 -> [_ w470]
            tunnel: ["" w467] -> w456
            frame False {
            }
            frame True {
              n193 = call "ASYNC_Adam_server.vi"("Values"=w471, "Channel Names"=w470) -> ("Scan Comments"=w468:string[])  [unwired: 1 in, 2 out]
              n194 = Index Array(array=w468, index=0) -> (element=w467:string)
            }
          }
        }
      }
      frame #15 {
        # "To automatically control the request for the University Stall chiller to run."
        n195 = while {
          tunnel: w476 -> [w484]
          tunnel: w475 -> [w485]
          shift-right: [w479] -> _
          shift-left: _ -> [w494]
          shift-left: _ -> [w493]
          shift-left: _ -> [w492]
          tunnel: [w478] -> w474
          tunnel: [w477] -> w473
          stop <- FALSE continue-if-true
          n196 = Build Array("EnFlo_Tunnel:Chiller_Pump:Enable" ("Desired Ch to Read"), "Aero_Tunnel:Cooling_Pump:Enable" ("Desired Ch to Read")) -> (w486:string[])
          n197 = call "Read_Earlier_Channels.vi"("Present scan array"=w484, "Ch names"=w485, "Desired Channels"=w486) -> ("Scan comments"=w477:string, "Index 0"=w483:dbl, "Index 1"=w482:dbl)  [unwired: 3 out]
          n198 = Build Array(w483, w482) -> (w481:dbl[])
          n199 = Greater?(x=w481, y=0.5) -> (0:w480:bool[])
          n200 = Or Array Elements(Boolean array=w480) -> (logical OR=w479:bool)
          n201 = Compound Arithmetic op=AND(w479, w494, invert w493, invert w492) -> (w490:bool)
          n202 = Compound Arithmetic op=AND(invert w479, invert w494, w493, w492) -> (w491:bool)
          n203 = Or(x=w490, y=w491) -> (x .or. y?=w489:bool)
          n204 = case shown="True" w489 {
            tunnel: w479 -> [_ w503]
            tunnel: [string[] [] ("Scan Comments") w498] -> w478
            frame False {
            }
            frame True {
              n205 = case shown="False" w503 {
                tunnel: [string[] ["University:Chilled Water:Requested"] ("Channel Names") string[] ["University:Chilled Water:Requested"] ("Channel Names")] -> w502
                tunnel: [1.0 ("y") 0.0 ("y")] -> w499
                frame True {
                }
                frame False {
                }
              }
              n206 = Array Size(array=w502) -> (size(s)=w500:i32)
              n207 = Initialize Array(w499, w500) -> (w501:dbl[])
              n208 = call "ASYNC_Adam_server.vi"("Values"=w501, "Channel Names"=w502) -> ("Scan Comments"=w498:string[])  [unwired: 1 in, 2 out]
            }
          }
        }
        n209 = Concatenate Strings(w474, w473) -> (w472:string)
      }
      frame #16 {
        # "Exercise the floor cooling valve once a week"
        n210 = while {
          shift-right: [w512] -> _
          shift-left: _ -> [w517]
          tunnel: w510 -> [w512]
          tunnel: w509 -> [w514]
          tunnel: [w511] -> w508
          stop <- TRUE stop-if-true
          n211 = Not Equal?(x=w512, y=w517) -> (x != y?=w515:bool)
          n212 = Compound Arithmetic op=AND(w515, w514) -> (w513:bool)
          n213 = case shown="True" w513 {
            tunnel: w512 -> [_ w524]
            tunnel: ["" w519] -> w511
            frame False {
            }
            frame True {
              n214 = Select(t=1.0, s=w524, f=0.0) -> (s? t:f=w525:dbl)
              n215 = Build Array(w525) -> (w528:dbl[])
              n216 = Build Array("EnFlo_Tunnel:Floor_Cooling:Enable") -> (w527:string[])
              n217 = call "ASYNC_Adam_server.vi"("Values"=w528, "Channel Names"=w527) -> ("Scan Comments"=w520:string[])  [unwired: 1 in, 2 out]
              n218 = Index Array(array=w520, index=0) -> (element=w519:string)
            }
          }
        }
      }
      frame #17 {
        w538 = "Status:of:"
        # "is any rig running?"
        # "Exercise UPS once a week to keep battery in good health provided no rigs are running"
        n219 = String Length(string=w538) -> (length=w539:i32)
        n220 = for {
          tunnel: w536 -> [w575] mode=indexing
          tunnel: w539 -> [w574]
          tunnel: w538 -> [w572]
          tunnel: w535 -> [w570] mode=indexing
          tunnel: [w569] -> w537 mode=indexing
          n221 = String Subset(string=w575, length (rest)=w574) -> (substring=w573:string)  [unwired: 1 out]
          n222 = Equal?(x=w572, y=w573) -> (x = y?=w571:bool)
          n223 = case shown="True" w571 {
            tunnel: w570 -> [_ w579]
            tunnel: [FALSE w577] -> w569
            frame False {
            }
            frame True {
              n224 = Less?(x=w579, y=4.0) -> (x < y?=w577:bool)
            }
          }
        }
        n225 = Or Array Elements(Boolean array=w537) -> (logical OR=w534:bool)
        n226 = Not(x=w534) -> (.not. x?=w533:bool)
        n227 = case shown="True" w533 {
          tunnel: [1.0 ("f") w555] -> w531
          frame False {
          }
          frame True {
            w560 = 2  # Minutes to switch off for
            n228 = Seconds To Date/Time() -> (date time rec=w564:T5)  [unwired: 2 out]
            n229 = Unbundle By Name(w564) -> ("day of week"=w567:i32, "hour"=w563:i32, "minute"=w561:i32)
            n230 = Less?(x=w561, y=w560) -> (x < y?=w557:bool)
            n231 = Equal?(x=2, y=w567) -> (x = y?=w559:bool)
            n232 = Equal?(x=w563, y=8) -> (x = y?=w558:bool)
            n233 = Compound Arithmetic op=AND(w559, w558, w557) -> (w556:bool)
            n234 = Select(t=0.0, s=w556, f=1.0) -> (s? t:f=w555:dbl)
          }
        }
        n235 = while {
          shift-right: [w545] -> _
          shift-left: _ -> [w546]
          tunnel: w531 -> [w545]
          tunnel: "ADAM:Server_PC:Enable" ("Desired Ch to Read") -> [w547]
          tunnel: w530 -> [w542]
          tunnel: [w540] -> w529
          stop <- TRUE stop-if-true
          n236 = Not Equal?(x=w545, y=w546) -> (x != y?=w543:bool)
          n237 = Compound Arithmetic op=OR(w543, invert w542) -> (w541:bool)
          n238 = Build Array(w547) -> (w548:string[])
          n239 = Build Array(w545) -> (w549:dbl[])
          n240 = case shown="False" w541 {
            tunnel: w549 -> [_ w553]
            tunnel: w548 -> [_ w552]
            tunnel: [string[] [] ("Scan Comments") w551] -> w540
            frame False {
            }
            frame True {
              n241 = call "ASYNC_Adam_server.vi"("Values"=w553, "Channel Names"=w552) -> ("Scan Comments"=w551:string[])  [unwired: 1 in, 2 out]
            }
          }
        }
      }
      frame #18 {
        n242 = Concatenate Strings(w583, w584, w585, w586, w587, w588, w589, w590, w597, w596, w595, w594, w593, w592, w591, w581, w580) -> (→"Scan comment":string)
      }
    }
  }
